vi "Receive Toveys.vi"(8 "error in (no error)":errorcluster, 11 "Model in":refnum<class "Model.lvclass">) -> (0 "error out":errorcluster, 3 "Model out":refnum<class "Model.lvclass">)   [LabVIEW 2015, in "Model.lvclass"]
uses:
  Model.lvclass
  Model.lvclass/Model.ctl
  TEI-9150/Tovey 9150.lvclass
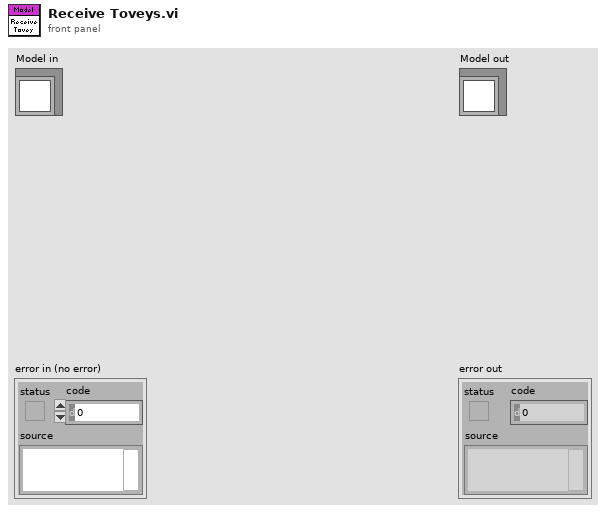
[diagram p1: front panel]
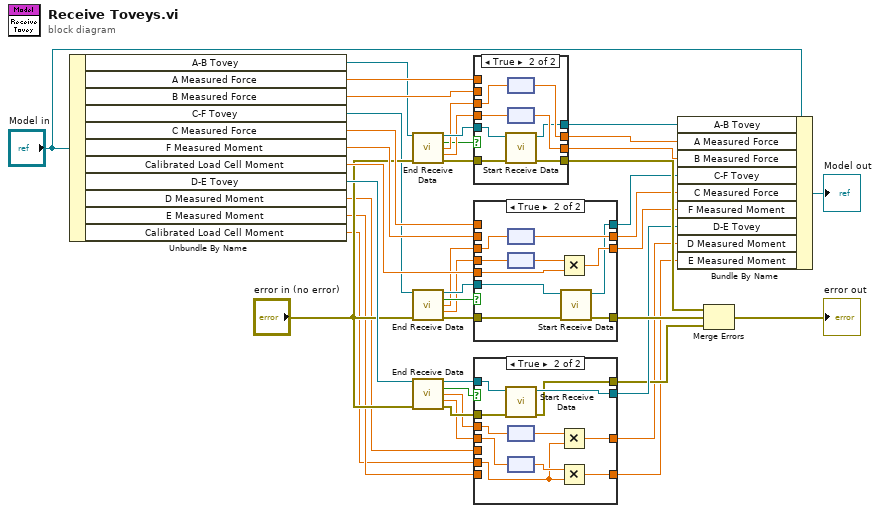
[diagram p0: block diagram]
diagram:
  n1 = Unbundle By Name("Model in") -> ("A-B Tovey"=w30:refnum<class "Tovey 9150.lvclass">, "A Measured Force"=w32:dbl[unit], "B Measured Force"=w31:dbl[unit], "C-F Tovey"=w1:refnum<class "Tovey 9150.lvclass">, "C Measured Force"=w23:dbl[unit], "F Measured Moment"=w22:dbl[unit], "Calibrated Load Cell Moment"=w21:dbl[unit], "D-E Tovey"=w13:refnum<class "Tovey 9150.lvclass">, "D Measured Moment"=w6:dbl[unit], "E Measured Moment"=w5:dbl[unit], "Calibrated Load Cell Moment"=w4:dbl[unit])
  n2 = call "End Receive Data.vi"("Tovey9150 in"=w30, "error in (no error)"="error in (no error)") -> ("Tovey9150 out"=w39:refnum<class "Tovey 9150.lvclass">, "Data Present"=w33:bool, "A"=w35:dbl, "B"=w34:dbl, "error out"=w36:errorcluster)  [unwired: 9 in]
  n3 = call "End Receive Data.vi"("Tovey9150 in"=w1, "error in (no error)"="error in (no error)") -> ("Tovey9150 out"=w27:refnum<class "Tovey 9150.lvclass">, "Data Present"=w20:bool, "A"=w19:dbl, "B"=w18:dbl, "error out"=w25:errorcluster)  [unwired: 9 in]
  n4 = call "End Receive Data.vi"("Tovey9150 in"=w13, "error in (no error)"="error in (no error)") -> ("Tovey9150 out"=w15:refnum<class "Tovey 9150.lvclass">, "Data Present"=w9:bool, "A"=w8:dbl, "B"=w7:dbl, "error out"=w11:errorcluster)  [unwired: 9 in]
  n5 = case shown="True" w33 {
    tunnel: w32 -> [w46 _]
    tunnel: [w46 w53] -> w29
    tunnel: w31 -> [w45 _]
    tunnel: [w45 w51] -> w28
    tunnel: w35 -> [_ w54]
    tunnel: w34 -> [_ w52]
    tunnel: w39 -> [w44 w50]
    tunnel: [w44 w49] -> w38
    tunnel: [w43 w48] -> w37
    tunnel: w36 -> [w43 w47]
    frame False {
    }
    frame True {
      n6 = call "Start Receive Data.vi"("error in (no error)"=w47, "Tovey9150 in"=w50) -> ("error out"=w48:errorcluster, "Tovey9150 out"=w49:refnum<class "Tovey 9150.lvclass">)  [unwired: 8 in]
      n7 = node(w54) -> (w53:dbl[unit])
      n8 = node(w52) -> (w51:dbl[unit])
    }
  }
  n9 = case shown="True" w20 {
    tunnel: w23 -> [w58 _]
    tunnel: [w58 w67] -> w17
    tunnel: w22 -> [w57 _]
    tunnel: [w57 w64] -> w16
    tunnel: w19 -> [_ w68]
    tunnel: w18 -> [_ w66]
    tunnel: w21 -> [_ w63]
    tunnel: w27 -> [w56 w62]
    tunnel: [w56 w61] -> w26
    tunnel: w25 -> [w55 w60]
    tunnel: [w55 w59] -> w24
    frame False {
    }
    frame True {
      n10 = node(w68) -> (w67:dbl[unit])
      n11 = node(w66) -> (w65:dbl[unit])
      n12 = Multiply(x=w65, y=w63) -> (x*y=w64:dbl[unit])
      n13 = call "Start Receive Data.vi"("error in (no error)"=w60, "Tovey9150 in"=w62) -> ("error out"=w59:errorcluster, "Tovey9150 out"=w61:refnum<class "Tovey 9150.lvclass">)  [unwired: 8 in]
    }
  }
  n14 = case shown="True" w9 {
    tunnel: w6 -> [w72 _]
    tunnel: [w72 w79] -> w3
    tunnel: w5 -> [w71 _]
    tunnel: [w71 w78] -> w2
    tunnel: w8 -> [_ w83]
    tunnel: w7 -> [_ w82]
    tunnel: w4 -> [_ w77]
    tunnel: w15 -> [w70 w76]
    tunnel: [w70 w75] -> w14
    tunnel: w11 -> [w69 w74]
    tunnel: [w69 w73] -> w10
    frame False {
    }
    frame True {
      n15 = call "Start Receive Data.vi"("error in (no error)"=w74, "Tovey9150 in"=w76) -> ("error out"=w73:errorcluster, "Tovey9150 out"=w75:refnum<class "Tovey 9150.lvclass">)  [unwired: 8 in]
      n16 = node(w83) -> (w80:dbl[unit])
      n17 = node(w82) -> (w81:dbl[unit])
      n18 = Multiply(x=w80, y=w77) -> (x*y=w79:dbl[unit])
      n19 = Multiply(x=w81, y=w77) -> (x*y=w78:dbl[unit])
    }
  }
  n20 = Bundle By Name(cluster="Model in", "A-B Tovey"=w38, "A Measured Force"=w29, "B Measured Force"=w28, "C-F Tovey"=w26, "C Measured Force"=w17, "F Measured Moment"=w16, "D-E Tovey"=w14, "D Measured Moment"=w3, "E Measured Moment"=w2) -> (→"Model out":refnum<class "Model.lvclass">)
  n21 = Merge Errors(w37, w24, w10) -> (→"error out":errorcluster)
